vi "双通道数据采集处理系统.vi"() -> ()   [LabVIEW 2012]
uses:
  <vilib>/measure/NI_MABase.lvlib
  <vilib>/Utility/file.llb/Write To Spreadsheet File (DBL).vi
panel:
  out "波形图表":dbl[][](graph)
  in  "通道2":u16(ring) items=["", "正弦波", "方波", "锯齿波", "三角波"]
  in  "系统退出":bool
  in  "数据回放":bool
  in  "数据记录":bool
  in  "采集数据":bool
  in  "F2":i16(knob) caption="Hz" scale=0.0..200.0
  in  "V2":i16(knob) scale=0.0..10.0
  in  "F1":i16(knob) caption="Hz" scale=0.0..200.0
  in  "电压基准":i16(knob) scale=2.0..10.0
  in  "V1":i16(knob) scale=0.0..10.0
  in  "时间基准":i16(knob) scale=3.0..30.0
  in  "通道1":u16(ring) items=["", "正弦波", "方波", "锯齿波", "三角波"]
  # "双通道数据采集处理系统"
  # "波形发生"
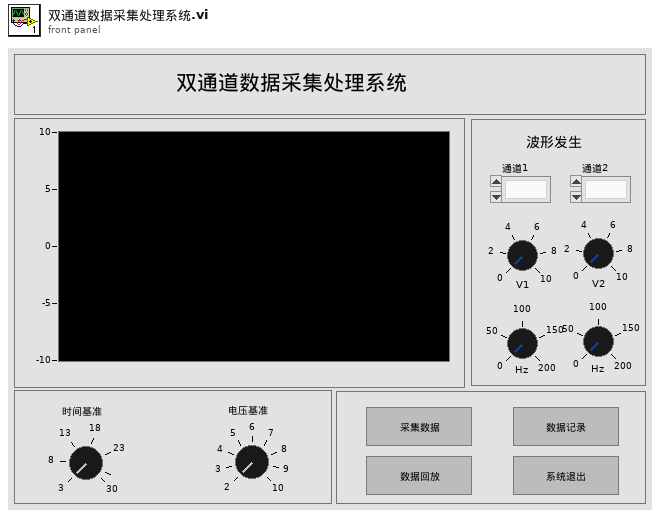
[diagram p1: front panel]
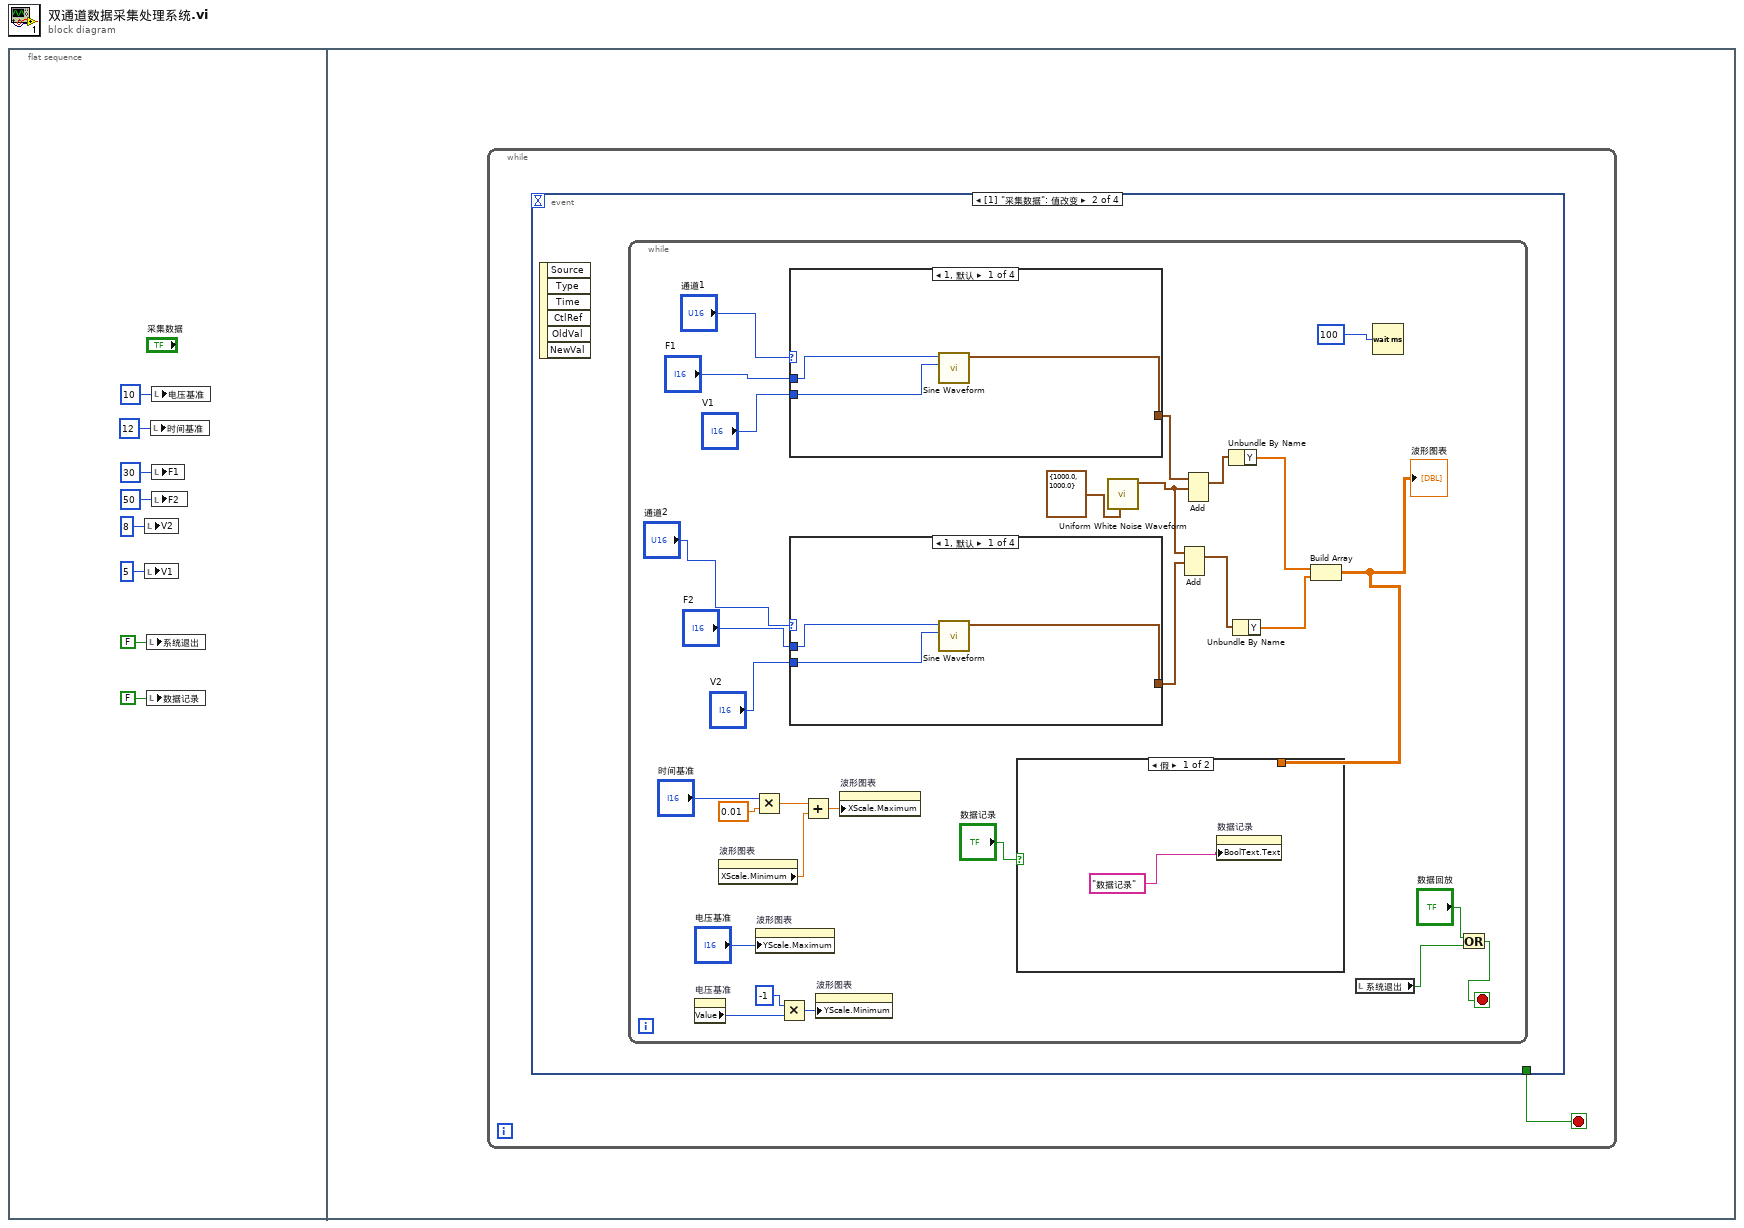
[diagram p0: block diagram]
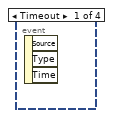
[diagram p2: hidden frame]
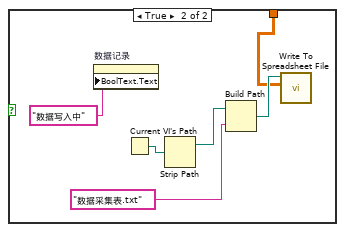
[diagram p3: hidden frame]
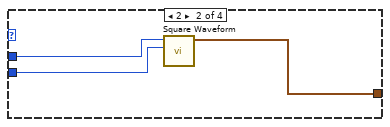
[diagram p4: hidden frame]
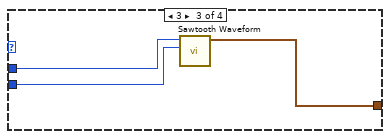
[diagram p5: hidden frame]
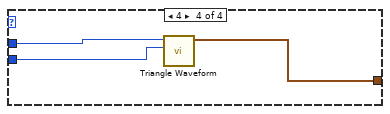
[diagram p6: hidden frame]
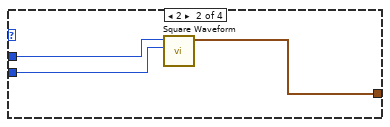
[diagram p7: hidden frame]
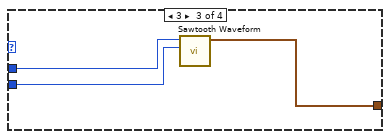
[diagram p8: hidden frame]
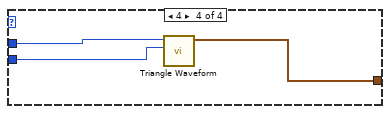
[diagram p9: hidden frame]
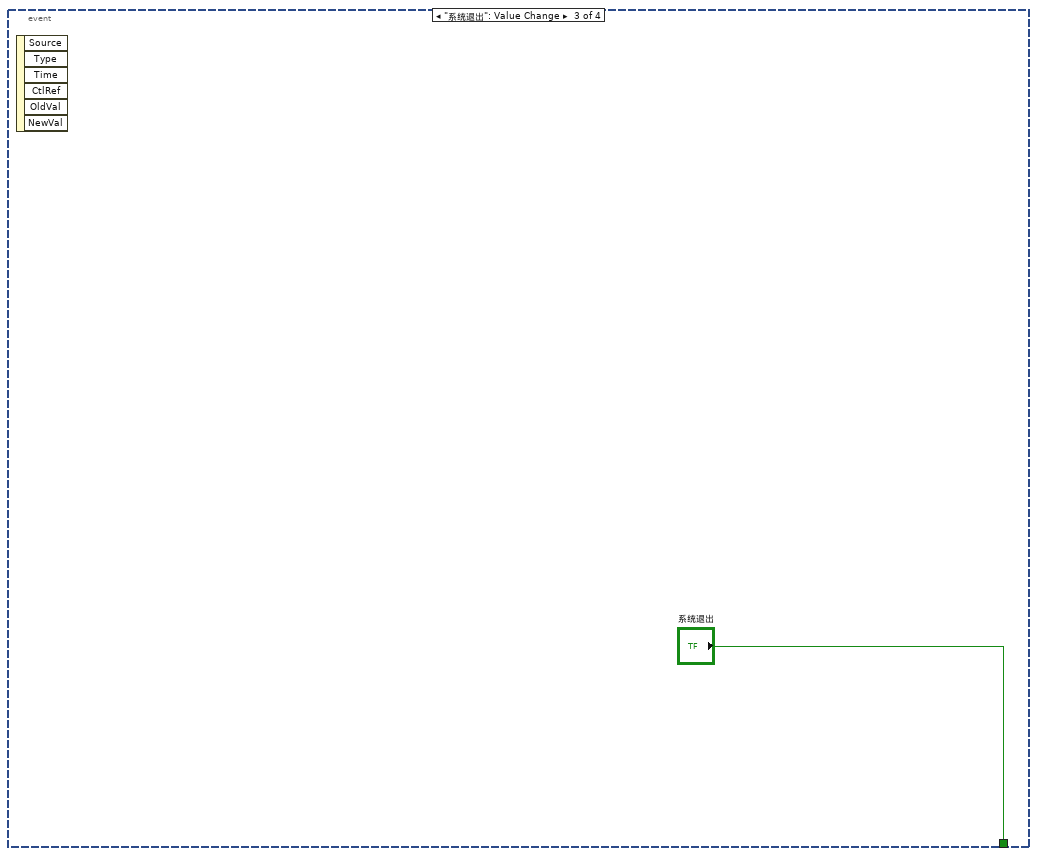
[diagram p10: hidden frame]
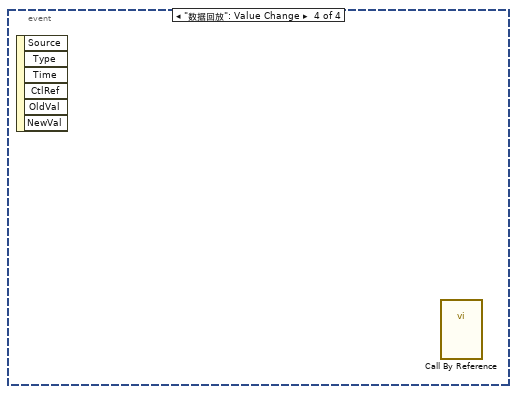
[diagram p11: hidden frame]
diagram:
  n1 = flat-sequence {
    frame #0 {
      n2 = local write "V2"(i16 8 ("V1")) -> ()
      n3 = local write "V1"(i16 5 ("V1")) -> ()
      n4 = local write "系统退出"(FALSE ("系统退出")) -> ()
      n5 = local write "数据记录"(FALSE ("数据记录")) -> ()
      n6 = local write "时间基准"(i16 12 ("V1")) -> ()
      n7 = local write "电压基准"(i16 10 ("V1")) -> ()
      n8 = local write "F1"(i16 30 ("V1")) -> ()
      n9 = local write "F2"(i16 50 ("V1")) -> ()
    }
    frame #1 {
      n10 = while {
        stop <- w9 stop-if-true
        n11 = event shown="[1] \"采集数据\": 值改变" {
          selector: _ -> [_ _ _ _]
          dyn-events: _ -> [_ _ _ _]
          timeout: _ -> [_ _ _ _]
          tunnel: [_ _ "系统退出" _] -> w9
          event Timeout {
            n12 = event-data() -> ()  [unwired: 1 in, 3 out]
          }
          event "采集数据": Value Change {
            n13 = event-data() -> ()  [unwired: 1 in, 6 out]
            n14 = while {
              stop <- w17 stop-if-true
              n15 = property on="电压基准" class="Knob (严格)"() -> ("Value"=w26:i16)  [unwired: 2 in, 2 out]
              n16 = property on="波形图表" class="WFChart (严格)"() -> ("XScale.Minimum"=w19:dbl)  [unwired: 2 in, 2 out]
              n17 = Multiply(x="时间基准", y=0.01) -> (x*y=w21:dbl)
              n18 = property on="波形图表" class="WFChart (严格)"("YScale.Maximum"="电压基准") -> ()  [unwired: 2 in, 2 out]
              n19 = Multiply(x=i16 -1, y=w26) -> (x*y=w24:i16)
              n20 = case shown="1, 默认" "通道1" {
                tunnel: [w60 w61 w64 w67] -> w15
                tunnel: "V1" -> [w59 w62 w65 w69]
                tunnel: "F1" -> [w58 w63 w66 w68]
                frame 1, Default {
                  n21 = call <vilib>:"Sine Waveform.vi"("amplitude"=w59, "frequency"=w58) -> ("signal out"=w60:waveform(dbl))  [unwired: 8 in, 1 out]
                }
                frame 2 {
                  n22 = call <vilib>:"Square Waveform.vi"("amplitude"=w62, "frequency"=w63) -> ("signal out"=w61:waveform(dbl))  [unwired: 8 in, 1 out]
                }
                frame 3 {
                  n23 = call <vilib>:"Sawtooth Waveform.vi"("amplitude"=w65, "frequency"=w66) -> ("signal out"=w64:waveform(dbl))  [unwired: 8 in, 1 out]
                }
                frame 4 {
                  n24 = call <vilib>:"Triangle Waveform.vi"("amplitude"=w69, "frequency"=w68) -> ("signal out"=w67:waveform(dbl))  [unwired: 8 in, 1 out]
                }
              }
              n25 = case shown="1, 默认" "通道2" {
                tunnel: [w48 w49 w52 w55] -> w14
                tunnel: "V2" -> [w47 w50 w53 w57]
                tunnel: "F2" -> [w46 w51 w54 w56]
                frame 1, Default {
                  n26 = call <vilib>:"Sine Waveform.vi"("amplitude"=w47, "frequency"=w46) -> ("signal out"=w48:waveform(dbl))  [unwired: 8 in, 1 out]
                }
                frame 2 {
                  n27 = call <vilib>:"Square Waveform.vi"("amplitude"=w50, "frequency"=w51) -> ("signal out"=w49:waveform(dbl))  [unwired: 8 in, 1 out]
                }
                frame 3 {
                  n28 = call <vilib>:"Sawtooth Waveform.vi"("amplitude"=w53, "frequency"=w54) -> ("signal out"=w52:waveform(dbl))  [unwired: 8 in, 1 out]
                }
                frame 4 {
                  n29 = call <vilib>:"Triangle Waveform.vi"("amplitude"=w57, "frequency"=w56) -> ("signal out"=w55:waveform(dbl))  [unwired: 8 in, 1 out]
                }
              }
              n30 = Add(x=w21, y=w19) -> (x+y=w20:dbl)
              n31 = property on="波形图表" class="WFChart (严格)"("YScale.Minimum"=w24) -> ()  [unwired: 2 in, 2 out]
              n32 = property on="波形图表" class="WFChart (严格)"("XScale.Maximum"=w20) -> ()  [unwired: 2 in, 2 out]
              n33 = call <vilib>:"Uniform White Noise Waveform.vi"("sampling info"=cluster{"Fs":dbl, "#s":dbl} {"Fs"=1000.0, "#s"=1000.0}) -> ("signal out"=w13:waveform(dbl))  [unwired: 9 in, 1 out]
              n34 = Add(1:w14, 2:w13) -> (0:w11:waveform(dbl))  [unwired: 1 in, 1 out]
              n35 = Add(1:w13, 2:w15) -> (0:w12:waveform(dbl))  [unwired: 1 in, 1 out]
              n36 = Unbundle By Name(w12) -> ("Y"=w32:dbl[])
              n37 = Unbundle By Name(w11) -> ("Y"=w31:dbl[])
              n38 = Build Array(w32, w31) -> (w29:dbl[][])
              "波形图表" <- w29
              n39 = case shown="假" "数据记录" {
                tunnel: w29 -> [_ w41]
                frame False {
                  n40 = property on="数据记录" class="Bool (严格)"("BoolText.Text"="数据记录" ("布尔文本.文本")) -> ()  [unwired: 2 in, 2 out]
                }
                frame True {
                  n41 = property on="数据记录" class="Bool (严格)"("BoolText.Text"="数据写入中" ("布尔文本.文本")) -> ()  [unwired: 2 in, 2 out]
                  n42 = Current VI's Path() -> (path=w45:path)
                  n43 = Strip Path(path=w45) -> (stripped path=w44:path)  [unwired: 1 out]
                  n44 = Build Path(base path=w44, name or relative path="数据采集表.txt") -> (appended path=w42:path)
                  n45 = call-poly <vilib>:"Write To Spreadsheet File.vi"("2D data"=w41, "file path (dialog if empty)"=w42) -> ()  [unwired: 6 in, 1 out]
                }
              }
              n46 = local read "系统退出"() -> (w16:bool)
              n47 = Wait (ms)(milliseconds to wait=u32 100 ("等待时间（毫秒）")) -> ()  [unwired: 1 out]
              n48 = Or(x="数据回放", y=w16) -> (x .or. y?=w17:bool)
            }
          }
          event "系统退出": Value Change {
            n49 = event-data() -> ()  [unwired: 1 in, 6 out]
          }
          event "数据回放": Value Change {
            n50 = event-data() -> ()  [unwired: 1 in, 6 out]
            n51 = call-by-ref "?"() -> ()  [unwired: 14 in, 2 out]
          }
        }
      }
    }
  }
